vi "실습 6-1 이벤트핸들러.vi"() -> ()   [LabVIEW 2014]
uses:
  <vilib>/Analysis/NI_AALBase.lvlib
panel:
  out "웨이브폼 그래프":dbl[](graph)
  in  "정지":bool
  in  "삼각 파형":bool
  in  "사인 파형":bool
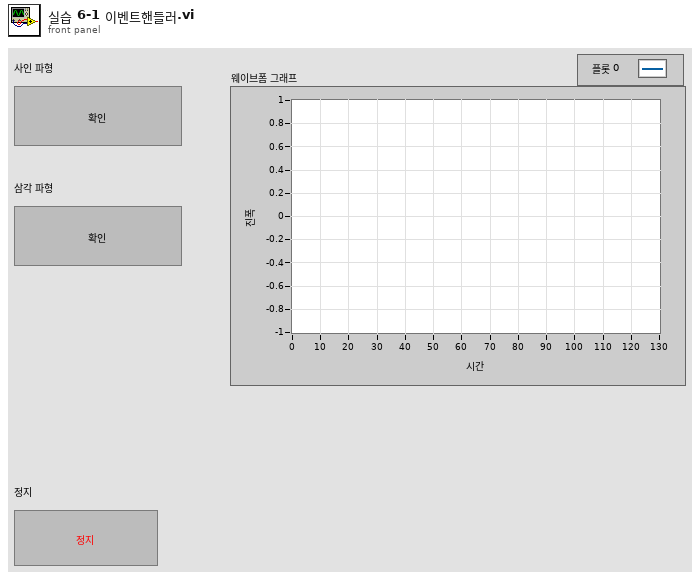
[diagram p1: front panel]
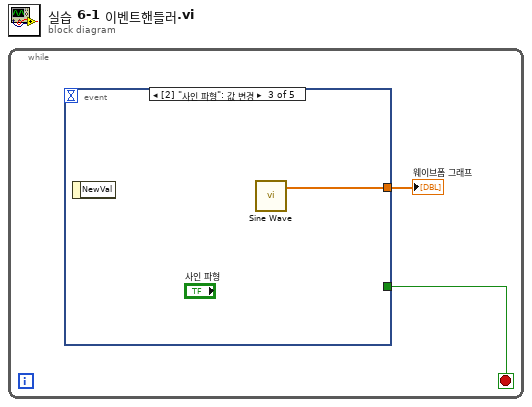
[diagram p0: block diagram]
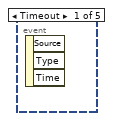
[diagram p2: hidden frame]
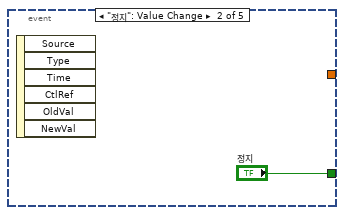
[diagram p3: hidden frame]
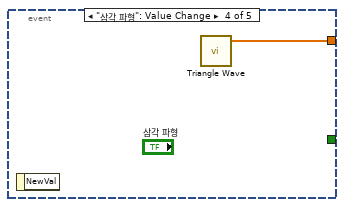
[diagram p4: hidden frame]
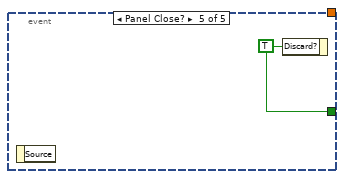
[diagram p5: hidden frame]
diagram:
  n1 = while {
    stop <- w2 stop-if-true
    n2 = event shown="[2] \"사인 파형\": 값 변경" {
      selector: _ -> [_ _ _ _ _]
      dyn-events: _ -> [_ _ _ _ _]
      timeout: _ -> [_ _ _ _ _]
      tunnel: [_ "정지" _ _ w6] -> w2
      tunnel: [_ _ w4 w5 _] -> w1
      event Timeout {
        n3 = event-data() -> ()  [unwired: 1 in, 3 out]
      }
      event "정지": Value Change {
        n4 = event-data() -> ()  [unwired: 1 in, 6 out]
      }
      event "사인 파형": Value Change {
        n5 = event-data() -> ()  [unwired: 1 in, 1 out]
        n6 = call <vilib>:"Sine Wave.vi"() -> ("sine wave"=w4:dbl[])  [unwired: 5 in, 2 out]
      }
      event "삼각 파형": Value Change {
        n7 = event-data() -> ()  [unwired: 1 in, 1 out]
        n8 = call <vilib>:"Triangle Wave.vi"() -> ("triangle wave"=w5:dbl[])  [unwired: 5 in, 2 out]
      }
      event Panel Close? {
        w6 = TRUE ("버림?")
        n9 = event-data() -> ()  [unwired: 1 in, 1 out]
        n10 = event-data("Discard?"=w6) -> ()  [unwired: 1 in, 1 out]
      }
    }
    "웨이브폼 그래프" <- w1
  }
